vi "update.assets.vi"(8 "error in (no error)":errorcluster, 10 "Assets":refnum<class "asset.lvclass">[](array[class]), 11 "Run in":refnum<class "Run.lvclass">) -> (0 "error out":errorcluster, 3 "Run out":refnum<class "Run.lvclass">)   [LabVIEW 2020, in "Run.lvclass"]
uses:
  Run.lvclass
  Nominal Client/Nominal Client.lvclass
  asset/asset.lvclass
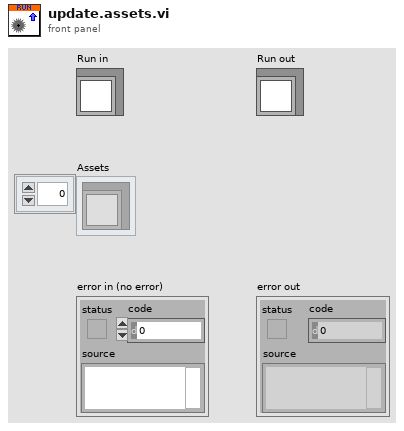
[diagram p1: front panel]
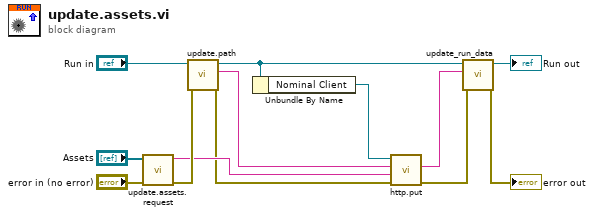
[diagram p0: block diagram]
diagram:
  n1 = call "update.assets.request.vi"("error in"="error in (no error)", "Assets"="Assets") -> ("error out"=w8:errorcluster, "request"=w7:string)  [unwired: 8 in]
  n2 = call "update.path.vi"("error in"=w8, "Run"="Run in") -> ("error out"=w6:errorcluster, "path"=w11:string, "Run Out"=w5:refnum<class "Run.lvclass">)  [unwired: 7 in]
  n3 = Unbundle By Name(w5) -> ("Nominal Client"=w12:refnum<class "Nominal Client.lvclass">)
  n4 = call "http.put.vi"("error in"=w6, "Body"=w7, "Path"=w11, "Nominal Client in"=w12) -> ("error out"=w2:errorcluster, "Response"=w3:string)  [unwired: 5 in, 1 out]
  n5 = call "update_run_data.vi"("error in"=w2, "Run JSON"=w3, "Run in"=w5) -> ("error out"=→"error out":errorcluster, "Run out"=→"Run out":refnum<class "Run.lvclass">)  [unwired: 7 in]
